vi "PH_gentec_Powermeter.Action Measure.vi"(0 "VI in":refnum<vi>, 5 "error in (no error)":errorcluster) -> (14 "VI out":refnum<vi>, 19 "error out":errorcluster)   [LabVIEW 2014, in "PH_gentec_Powermeter.lvlib"]
uses:
  PH_gentec_Powermeter.lvlib
  PH_Powermeter_BaseClass/PH_Powermeter_BaseClass.lvlib
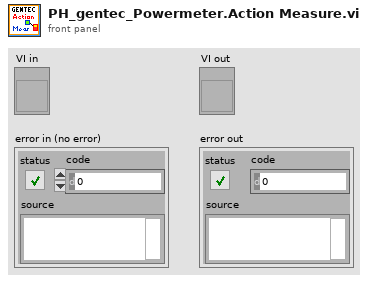
[diagram p1: front panel]
types:
  T1 = typedef "PH_Powermeter_BaseClass.lvlib/PH_Powermeter_BaseClass.i attribute.ctl" = cluster{"GUI References":T2, "Connection":T3, "Head Attributes":T5, "VISA resource":refnum<visa-resource-name>, "Energy":T6, "Service ID Energy":i32, "Wanted Settings":T7, "Current Settings":T7}
  T2 = typedef "PH_Powermeter_BaseClass.lvlib/PH_Powermeter_BaseClass.GUI Refs.ctl" = cluster{"Head Attributes":refnum<vi>, "Energy":refnum<vi>, "Connection":refnum<vi>, "VISA Resource":refnum<vi>, "Energy evolution":refnum<vi>, "Scaling Factor":refnum<vi>, "Range":refnum<vi>, "Wavelength":refnum<vi>, "Trigger Level":refnum<vi>, "Wanted Settings":refnum<vi>, "Current Settings":refnum<vi>}
  T3 = typedef "PH_Powermeter_BaseClass.lvlib/PH_Powermeter_BaseClass.Connection.ctl" = cluster{"failed checks":i8, "Timeout":bool, "Data read":string, "Failure":bool, "Error":bool, "State":T4}
  T4 = typedef "PH_Powermeter_BaseClass.lvlib/PH_Powermeter_BaseClass.State.ctl" = enum32{"off", "operating", "opened", "checked", "connected", "Sets to change", "running"}
  T5 = typedef "PH_Powermeter_BaseClass.lvlib/PH_Powermeter_BaseClass.Head Attributes.ctl" = cluster{"Instrument Type":string, "Head Version":string, "Head Name":string, "Serial Number":string, "Firmware":string, "Sensor Type":string, "MinimumRange":u32, "Maximum Range":u32, "Min Wavelength":i32, "Max Wavelength":i32}
  T6 = typedef "PH_Powermeter_BaseClass.lvlib/PH_Powermeter_BaseClass.Energy.ctl" = cluster{"current Value":dbl, "unscaled":dbl, "Scaling Factor":dbl}
  T7 = typedef "PH_Powermeter_BaseClass.lvlib/PH_gentec_BaseClass.Head Settings.ctl" = cluster{"Trigger Level":dbl, "Wavelength":u32, "Range":u32}
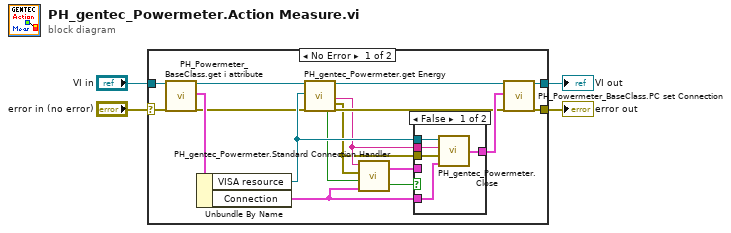
[diagram p0: block diagram]
diagram:
  n1 = case shown="No Error" "error in (no error)" {
    selector: "error in (no error)" -> [w6 w28]
    tunnel: [w16 w28] -> w1
    tunnel: [w15 w29] -> w2
    tunnel: "VI in" -> [w8 w29]
    frame No Error {
      n2 = call "PH_Powermeter_BaseClass.get i attribute.vi"("i ref in"=w8, "error in (no error)"=w6) -> ("i ref out"=w7:refnum<vi>, "i attribute"=w21:T1, "error out"=w5:errorcluster)  [unwired: 15 in]
      n3 = Unbundle By Name(w21) -> ("VISA resource"=w20:refnum<visa-resource-name>, "Connection"=w14:T3)
      n4 = call "PH_gentec_Powermeter.get Energy.vi"("i ref in"=w7, "VISA resource in"=w20, "error in"=w5) -> ("Timeout"=w13:bool, "i ref out"=w18:refnum<vi>, "Error Message"=w11:string, "Device Error out"=w10:errorcluster, "error out"=w17:errorcluster)  [unwired: 12 in]
      n5 = call "PH_gentec_Powermeter.Standard Connection Handler.vi"("Connection in"=w14, "Timeout"=w13, "Device Error"=w10, "Error"=w11) -> ("No problem"=w9:bool, "Connection out"=w12:T3)
      n6 = case shown="False" w9 {
        tunnel: w20 -> [w26 _]
        tunnel: [w25 w27] -> w19
        tunnel: w12 -> [_ w27]
        tunnel: w11 -> [w24 _]
        tunnel: w10 -> [w23 _]
        tunnel: w14 -> [w22 _]
        frame False {
          n7 = call "PH_gentec_Powermeter.Close.vi"("Connection in"=w22, "Device Error in"=w23, "Error Message"=w24, "VISA Refnum in"=w26) -> ("Connection out"=w25:T3)
        }
        frame True {
        }
      }
      n8 = call "PH_Powermeter_BaseClass.PC set Connection.vi"("VI in"=w18, "Connection"=w19, "error in (no error)"=w17) -> ("VI out"=w15:refnum<vi>, "error out"=w16:errorcluster)  [unwired: 15 in]
    }
    frame Error {
    }
  }
  "VI out" <- w2
  "error out" <- w1
